vi "Vision Research Phantom Series PhFile PhEnableCineColor.vi"(0 "CH in":u32=1, 5 "Error In (no error)":errorcluster, 8 "Simulate? (False)":bool) -> (14 "CH out":u32=1, 19 "Error Out":errorcluster)   [LabVIEW 2013, in "VRI.lvlib"]
doc: "PhFile.dll\n\nPhEnableCineColor\nEXIMPROC HRESULT PhEnableCineColor(CINEHANDLE CH, BOOL bEnableColor);\n\nParameters Description\nCH(in) Handle of the cine.\nbEnableColor(in) TRUE to activate color interpolation for the cine images.\n FALSE to deactivate it.\nReturn HRESULT (0=Ok)\nComments Activates/Deactivates color interpolation for the cine. \n This operation changes the cine's BITMAPINFOHEADER.\n Call PhGetCineBMIH to get the new BITMAPINFOHEADER."
uses:
  VRI.lvlib
  Projects/SDK/32-bit/Vision Research Phantom Series Labview Driver/Phantom DLLs/PhFile.dll
panel:
  in  "bEnableColor in":bool
  # "For instructions on the use of this VI, press Ctrl+H to display the help window and move the mouse over the icon, controls, and indicators"
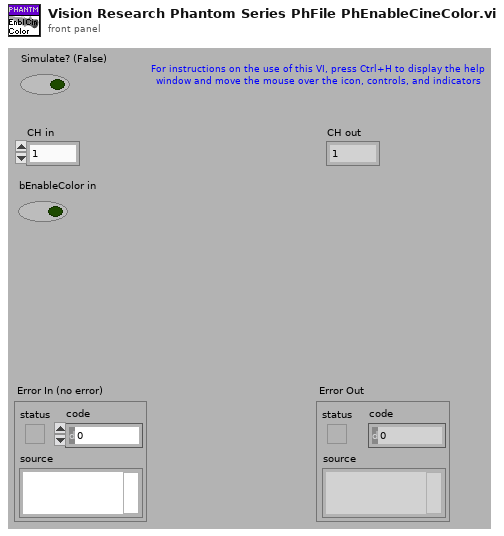
[diagram p1: front panel]
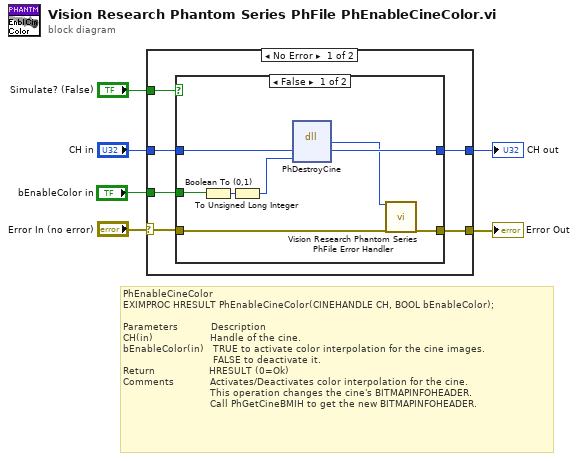
[diagram p0: block diagram]
diagram:
  # "PhEnableCineColor\nEXIMPROC HRESULT PhEnableCineColor(CINEHANDLE CH, BOOL bEnableColor);\n\nParameters           Description\nCH(in)                   Handle of the cine.\nbEnableColor(in)   TRUE to activate color interpolation for the cine images.\n                              FALSE to deactivate it.\nReturn                  HRESULT (0=Ok)\nComments            Activates/Deactivates color interpolation for the cine. \n                             This operation changes the cine's BITMAPINFOHEADER.\n                             Call PhGetCineBMIH to get the new BITMAPINFOHEADER."
  n1 = case shown="No Error" "Error In (no error)" {
    selector: "Error In (no error)" -> [w12 w24]
    tunnel: [w11 w24] -> w5
    tunnel: "Simulate? (False)" -> [w10 _]
    tunnel: "CH in" -> [w9 w23]
    tunnel: [w8 w23] -> w2
    tunnel: "bEnableColor in" -> [w7 _]
    frame No Error {
      n2 = case shown="False" w10 {
        tunnel: w12 -> [w19 w22]
        tunnel: [w20 w22] -> w11
        tunnel: w9 -> [w18 w21]
        tunnel: [w17 w21] -> w8
        tunnel: w7 -> [w14 _]
        frame False {
          n3 = Boolean To (0,1)(Boolean=w14) -> (0, 1=w15:i16)
          n4 = To Unsigned Long Integer(number=w15) -> (unsigned 32bit integer=w13:u32)
          n5 = dll-call lib="C:/Projects/SDK/32-bit/Vision Research Phantom Series Labview Driver/Phantom DLLs/PhFile.dll" fn="PhDestroyCine"("CH"=w18, "bEnableColor"=w13) -> ("HRESULT"=w16:i32, "CH"=w17:u32)  [unwired: 4 in, 2 out]
          n6 = call "Vision Research Phantom Series PhFile Error Handler.vi"("Error Code (0)"=w16, "Error In (no error)"=w19) -> ("Error Out"=w20:errorcluster)  [unwired: 17 out]
        }
        frame True {
          # "It looks as though the dlls can provide simulated data so this case may not have to be used"
        }
      }
    }
    frame Error {
    }
  }
  "Error Out" <- w5
  "CH out" <- w2
